vi "assignment1_2.vi"() -> ()   [LabVIEW 2014]
doc: "A dice rolling game with two players which stops when user pushes the stop button. Time delay can be used to slow the game down."
panel:
  out "P2 average":dbl
  out "P1 average":dbl
  out "?":dbl
  out "?":dbl
  out "?":dbl
  out "?":dbl
  out "?":dbl
  out "?":dbl
  out "?":dbl
  out "?":dbl
  out "?":dbl
  out "?":dbl
  out "tie rate":dbl
  out "P2 win rate":dbl
  out "P1 win rate":dbl
  out "Win Rate Chart":cluster{dbl, dbl, dbl}(graph)
  out "result":string
  in  "Roll Button":bool
  # "P1"
  # "P2"
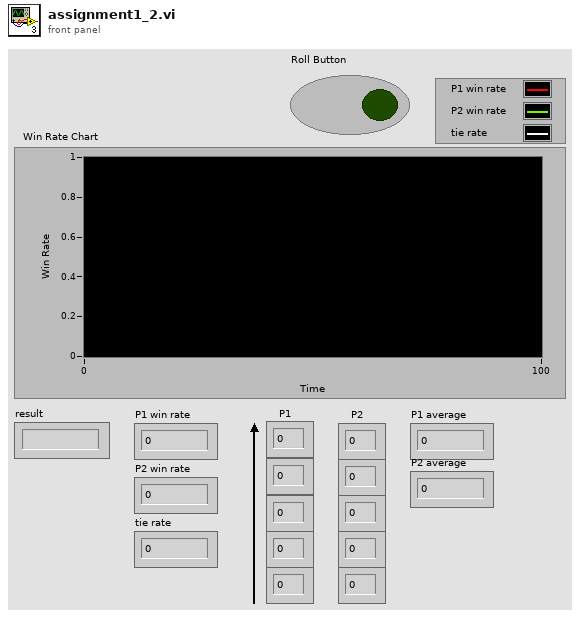
[diagram p1: front panel]
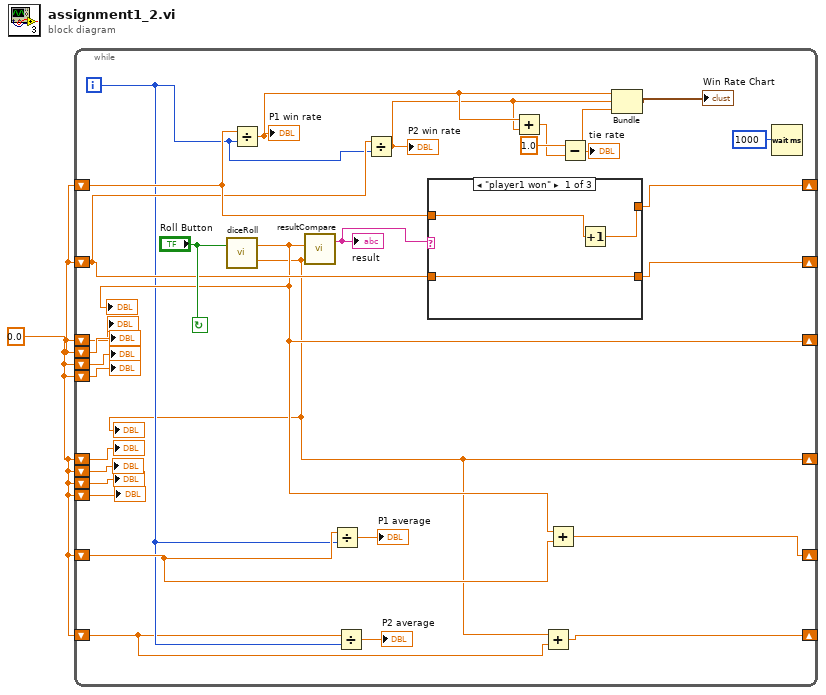
[diagram p0: block diagram]
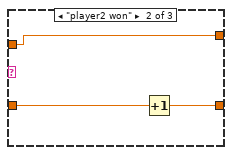
[diagram p2: hidden frame]
diagram:
  w1 = 0.0
  n1 = while {
    shift-right: [w28] -> _
    shift-left: w1 -> [w27]
    shift-right: [w26] -> _
    shift-left: w1 -> [w25]
    shift-right: [w10] -> _
    shift-left: w1 -> [w12]
    shift-left: w1 -> [w15]
    shift-left: w1 -> [w14]
    shift-left: w1 -> [w13]
    shift-right: [w4] -> _
    shift-left: w1 -> [w11]
    shift-left: w1 -> [w16]
    shift-left: w1 -> [w17]
    shift-left: w1 -> [w18]
    shift-right: [w8] -> _
    shift-left: w1 -> [w7]
    shift-right: [w2] -> _
    shift-left: w1 -> [w3]
    i -> [w6]
    stop <- "Roll Button" continue-if-true
    n2 = call "diceRoll.vi"("Roll Button"="Roll Button") -> ("player2"=w4:dbl, "player1"=w10:dbl)  [unwired: 1 in]
    "?" <- w10
    "?" <- w4
    n3 = Divide(x=w27, y=w6) -> (x/y=w23:dbl)
    "P1 win rate" <- w23
    n4 = call "resultCompare.vi"("P2"=w4, "P1"=w10) -> ("result"=w29:string)  [unwired: 2 in]
    "result" <- w29
    n5 = Divide(x=w7, y=w6) -> (x/y=→"P1 average":dbl)
    n6 = Divide(x=w3, y=w6) -> (x/y=→"P2 average":dbl)
    n7 = Divide(x=w25, y=w6) -> (x/y=w22:dbl)
    "P2 win rate" <- w22
    n8 = case shown="\"player1 won\"" w29 {
      tunnel: [w34 w35 w39] -> w28
      tunnel: w27 -> [w33 w35 w39]
      tunnel: [w32 w36 w38] -> w26
      tunnel: w25 -> [w32 w37 w38]
      frame "player1 won" {
        n9 = Increment(x=w33) -> (x+1=w34:dbl)
      }
      frame "player2 won" {
        n10 = Increment(x=w37) -> (x+1=w36:dbl)
      }
      frame "tie", Default {
      }
    }
    n11 = Add(x=w23, y=w22) -> (x+y=w21:dbl)
    n12 = Add(x=w4, y=w3) -> (x+y=w2:dbl)
    n13 = Add(x=w10, y=w7) -> (x+y=w8:dbl)
    n14 = Subtract(x=1.0, y=w21) -> (x-y=w19:dbl)
    "tie rate" <- w19
    n15 = Bundle(w23, w22, w19) -> (→"Win Rate Chart":cluster{dbl, dbl, dbl})  [unwired: 1 in]
    n16 = Wait (ms)(milliseconds to wait=1000) -> ()  [unwired: 1 out]
    "?" <- w18
    "?" <- w15
    "?" <- w16
    "?" <- w17
    "?" <- w13
    "?" <- w14
    "?" <- w12
    "?" <- w11
  }
